vi "test Adjust Text to Fit Rectangle for Single Line.vi"(11 "Test Case In":refnum<class "test Adjust Text to Fit Rectangle.lvclass">) -> (0 "error out":errorcluster, 3 "Test Case Out":refnum<class "test Adjust Text to Fit Rectangle.lvclass">)   [LabVIEW 2020, in "test Adjust Text to Fit Rectangle.lvclass"]
uses:
  test Adjust Text to Fit Rectangle.lvclass
  C:/Program Files/National Instruments/LabVIEW 2026/vi.lib/Astemes/LUnit/Test Case.lvclass
  <vilib>/Astemes/LUnit/Test Case.lvclass/Test Case.ctl
  test Adjust Text to Fit Rectangle.lvclass/test Adjust Text to Fit Rectangle.ctl
  C:/Program Files/National Instruments/LabVIEW 2026/vi.lib/Astemes/LUnit/LUnit Runnable.lvclass
  D:/git/Silly-Billy/tests/test Adjust Text to Fit Rectangle/test Adjust Text to Fit Rectangle.lvclass
  <vilib>/LabVIEW Icon API/API_Text.ctl
  <vilib>/LabVIEW Icon API/LabVIEW Icon API.lvlib
  <vilib>/LabVIEW Icon API/Set Text Icon/Text-Based VI Icon.lvlib
  <vilib>/LabVIEW Icon API/API_Text Colors.ctl
  <vilib>/LabVIEW Icon API/lv_icon/Controls/Alignment.ctl
  <vilib>/LabVIEW Icon API/API_Test Settings.ctl
  <vilib>/Astemes/LUnit/Test Case.lvclass
panel:
  out "NOKs":T1[](array[typedef])
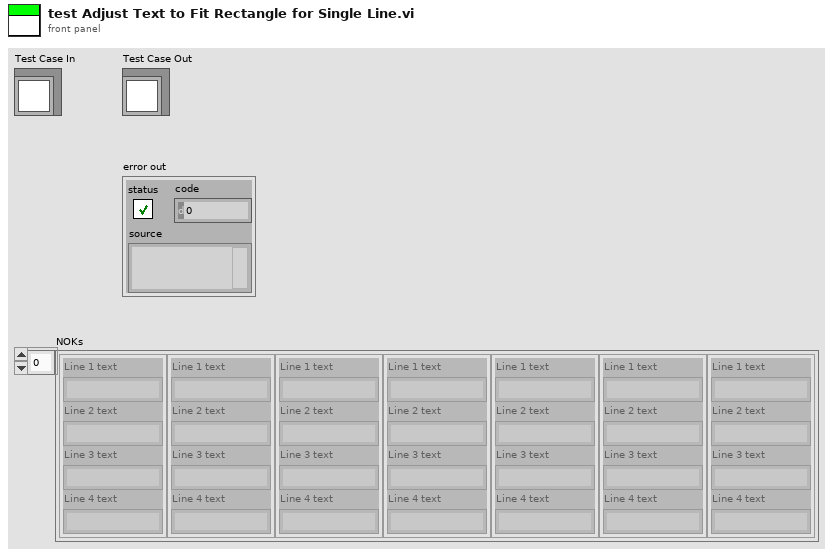
[diagram p1: front panel]
types:
  T1 = typedef "LabVIEW Icon API.lvlib/API_Text.ctl" = cluster{"Line 1 text":string, "Line 2 text":string, "Line 3 text":string, "Line 4 text":string}
  T2 = typedef "LabVIEW Icon API.lvlib/API_Test Settings.ctl" = cluster{"Font":string, "Alignment":T3, "Size":u8, "Center text":bool, "Capitalize text":bool, "Text color":T4}
  T3 = typedef "Alignment.ctl" = u16
  T4 = typedef "LabVIEW Icon API.lvlib/API_Text Colors.ctl" = cluster{"Line 1 color":u32, "Line 2 color":u32, "Line 3 color":u32, "Line 4 color":u32}
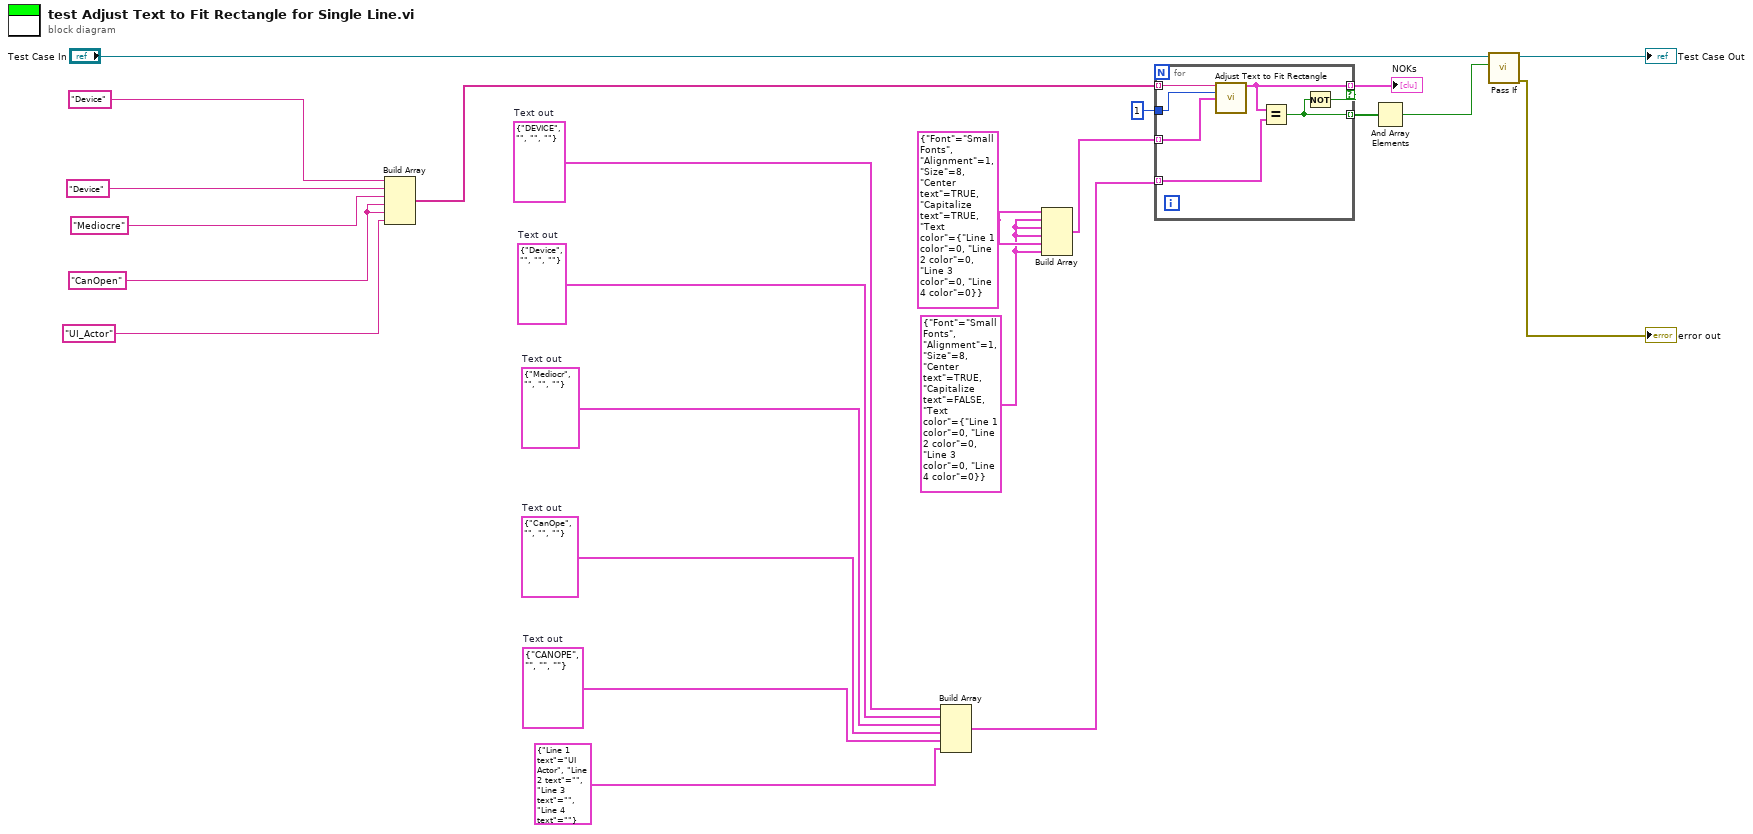
[diagram p0: block diagram]
diagram:
  w6 = T1 {"Line 1 text"="CANOPE", "Line 2 text"="", "Line 3 text"="", "Line 4 text"=""}  # Text out
  w8 = T1 {"Line 1 text"="CanOpe", "Line 2 text"="", "Line 3 text"="", "Line 4 text"=""}  # Text out
  w7 = "CanOpen" ("element")
  w2 = T2 {"Font"="Small Fonts", "Alignment"=1, "Size"=8, "Center text"=TRUE, "Capitalize text"=FALSE, "Text color"={"Line 1 color"=0, "Line 2 color"=0, "Line 3 color"=0, "Line 4 color"=0}} ("Text settings")
  w9 = T1 {"Line 1 text"="Mediocr", "Line 2 text"="", "Line 3 text"="", "Line 4 text"=""}  # Text out
  w11 = T1 {"Line 1 text"="Device", "Line 2 text"="", "Line 3 text"="", "Line 4 text"=""}  # Text out
  w5 = T2 {"Font"="Small Fonts", "Alignment"=1, "Size"=8, "Center text"=TRUE, "Capitalize text"=TRUE, "Text color"={"Line 1 color"=0, "Line 2 color"=0, "Line 3 color"=0, "Line 4 color"=0}} ("Text settings")
  w19 = T1 {"Line 1 text"="DEVICE", "Line 2 text"="", "Line 3 text"="", "Line 4 text"=""}  # Text out
  n1 = Build Array("Device" ("Input"), "Device" ("element"), "Mediocre" ("Input"), w7, w7, "UI_Actor" ("element")) -> (w18:string[])
  n2 = Build Array(w19, w11, w9, w8, w6, T1 {"Line 1 text"="UI Actor", "Line 2 text"="", "Line 3 text"="", "Line 4 text"=""} ("element")) -> (w16:T1[])
  n3 = Build Array(w5, w2, w2, w2, w5, w2) -> (w12:T2[])
  n4 = for {
    tunnel: w18 -> [w30] mode=indexing
    tunnel: 1 ("Number of Rows") -> [w29]
    tunnel: w12 -> [w28] mode=indexing
    tunnel: w16 -> [w27] mode=indexing
    tunnel: [w24] -> w15 mode=indexing
    tunnel: [w26] -> w1 mode=indexing if=w25
    n5 = call "Adjust Text to Fit Rectangle.vi"("VI Name"=w30, "Number of Rows"=w29, "Text settings"=w28) -> ("Text out"=w26:T1)  [unwired: 12 in]
    n6 = Equal?(x=w26, y=w27) -> (x = y?=w24:bool)
    n7 = Not(x=w24) -> (.not. x?=w25:bool)
  }
  "NOKs" <- w1
  n8 = And Array Elements(Boolean array=w15) -> (logical AND=w14:bool)
  n9 = call <vilib>:"Pass If.vi"("Pass?"=w14, "LUnit Test Case In"="Test Case In") -> ("error out"=→"error out":errorcluster, "LUnit Test Case Out"=→"Test Case Out":refnum<class "test Adjust Text to Fit Rectangle.lvclass">)  [unwired: 8 in]
